vi "arduinoInitValves.vi"(0 "valve open time":u32=1000) -> ()   [LabVIEW 2012]
uses:
  GlobalValves.vi
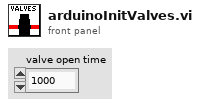
[diagram p1: front panel]
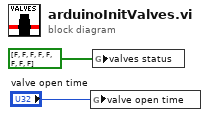
[diagram p0: block diagram]
diagram:
  n1 = global write "GlobalValves.vi" "valve open time"("valve open time") -> ()
  n2 = global write "GlobalValves.vi" "valves status"(bool[] [FALSE, FALSE, FALSE, FALSE, FALSE, FALSE, FALSE, FALSE] ("valve close 3")) -> ()
